vi "Set started from.vi"(8 "error in (no error)":errorcluster, 10 "started by tomo?":bool, 11 "ImageStack in":refnum<class "Invivo_ImageStack.lvclass">) -> (0 "error out":errorcluster, 3 "ImageStack out":refnum<class "Invivo_ImageStack.lvclass">)   [LabVIEW 2012, in "Invivo_ImageStack.lvclass"]
uses:
  Invivo_ImageStack.lvclass
  Invivo_ImageStack.lvclass/Invivo_ImageStack.ctl
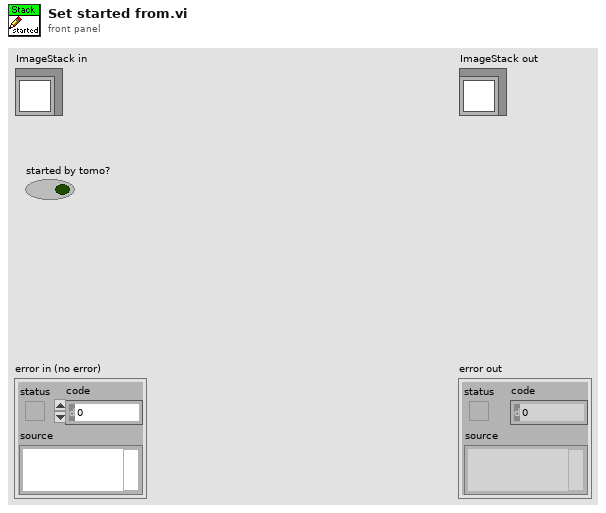
[diagram p1: front panel]
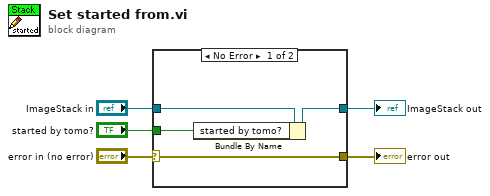
[diagram p0: block diagram]
diagram:
  n1 = case shown="No Error" "error in (no error)" {
    selector: "error in (no error)" -> [w9 w11]
    tunnel: [w9 w11] -> w4
    tunnel: [w7 w10] -> w2
    tunnel: "ImageStack in" -> [w8 w10]
    tunnel: "started by tomo?" -> [w6 _]
    frame No Error {
      n2 = Bundle By Name(cluster=w8, "started by tomo?"=w6) -> (w7:refnum<class "Invivo_ImageStack.lvclass">)
    }
    frame Error {
    }
  }
  "error out" <- w4
  "ImageStack out" <- w2
